vi "NF87XX.get start velocity.vi"(0 "i ref in":refnum<vi>, 2 "System":string="N/A", 5 "error in (no error)":errorcluster) -> (14 "i ref out":refnum<vi>, 16 "start velocity Mot 0 [Steps/s]":dbl, 17 "start velocity Mot 1 [Steps/s]":dbl, 18 "start velocity Mot 2 [Steps/s]":dbl, 19 "error out":errorcluster)   [LabVIEW 2014, in "NF87XX.lvlib"]
doc: "Gets the start velocity for all systems (drivers) and writes it to own attributes. Returns the start velocity of up to 3 motors in steps/s if \"System\" is found to be one of the driver names. Thereby 99999 indicates that an error occured or the value is not available.\n\nauthor: Stefan Götte\ndata: 09-JAN-2007\n\n\n\n\nLicense Agreement for this software:\n\nCopyright (C)\nGesellschaft für Schwerionenforschung, GSI\nPlanckstr. 1\n64291 Darmstadt\nGermany\n\nContact: D.Beck@gsi.de \n\nThis program is free software; you can redistribute it and/or modify it under the terms of the GNU General Public License as published by the Free Software Foundation; either version 2 of the license, or (at your option) any later version.\n\nThis program is distributed in the hope that it will be useful, but WITHOUT ANY WARRANTY; without even the implied warranty of MERCHANTABILITY or FITNESS FOR A PARTICULAR PURPOSE. See the GNU General License for more details (http://www.gnu.org).\n\nGesellschaft für Schwerionenforschung, GSI\nPlanckstr. 1, 64291 Darmstadt, Germany\nFor all questions and ideas contact: M.Richter@gsi.de, H.Brand@gsi.de or D.Beck@gsi.de.\nLast update: 17-JUN-2004"
uses:
  NF87XX.lvlib
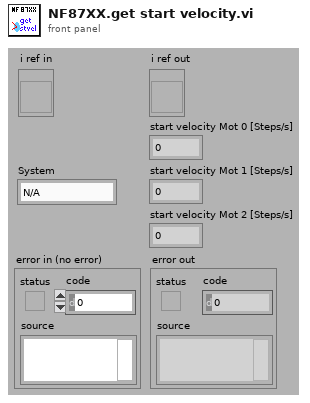
[diagram p1: front panel]
types:
  T1 = enum16{"User....", "DEF", "DIAG", "INI", "LOCK", "UNLOCK", "MAP", "SAV", "VER", "ACC", "CHL", "FOR", "GO", "HAL", "MOF", "MON", "MPV", "POS", "REL", "REV", "STA", "STO", "TYP", "VEL", "ABS", "SER", "NOS", "DRT", "FLI", "RLI", "FIN", "RIN", "AIN", "IN", "JOF", "JON", "OUT", "RES FINE", "RES COARSE", "02 (HEX)", "PWM", "CNT", "TMR", "HOSTNAME", "IPADDR", "IPMODE", "NETMASK", "GATEWAY", "DNSSRVR", "PASSWD", "ECHO", "MACADDR"}
  T2 = typedef "NF87XX.lvlib/NF87XX.driver Type.ctl" = enum16{"not defined", "3-ch open loop drv", "1-ch closed loop drv"}
  T3 = typedef "NF87XX.lvlib/NF87XX.i attribute.ctl" = cluster{"Con Settings":T4, "Drivers":T5[], "Status":cluster{"Service ID":i32, "Status":T7}, "Joystick available":bool, "VISA Resource":string}
  T4 = typedef "NewFocusPico - Driver np.lvlib/VISA & TCPIP Control.ctl" = cluster{"VISA or TCP/IP":bool, "Init Connection":bool, "Close Connection":bool, "Resource Name":refnum<visa-resource-name>, "hostname":string, "connection ID":refnum<k5>}
  T5 = typedef "NF87XX.lvlib/NF87XX.driver Settings.ctl" = cluster{"Name":string, "Driver Type":T2, "Pico Parameter type":T6, "Acceleration [Steps/s²]":cluster{"Motor 0":dbl, "Motor 1":dbl, "Motor 2":dbl}, "Start Velocity [Steps/s]":cluster{"Motor 0":dbl, "Motor 1":dbl, "Motor 2":dbl}, "Velocity [Steps/s]":cluster{"Motor 0":dbl, "Motor 1":dbl, "Motor 2":dbl}, "axis channel":i32, "Position":i32, "Position Service ID":i32}
  T6 = typedef "NewFocusPico - Driver np.lvlib/Pico Parameters.ctl" = cluster{"Pico Type":enum16{"Open-Loop Pico", "Close-Loop Pico", "Pico Ultra"}, "Acceleration (steps/sec^2)":string, "Velocity ( Hz)":string, "Driver":string, "Motor":string, "Channel":string, "Process Step":string}
  T7 = typedef "PH_StatusHandler.lvlib/PH_StatusHandler.Status.ctl" = i16
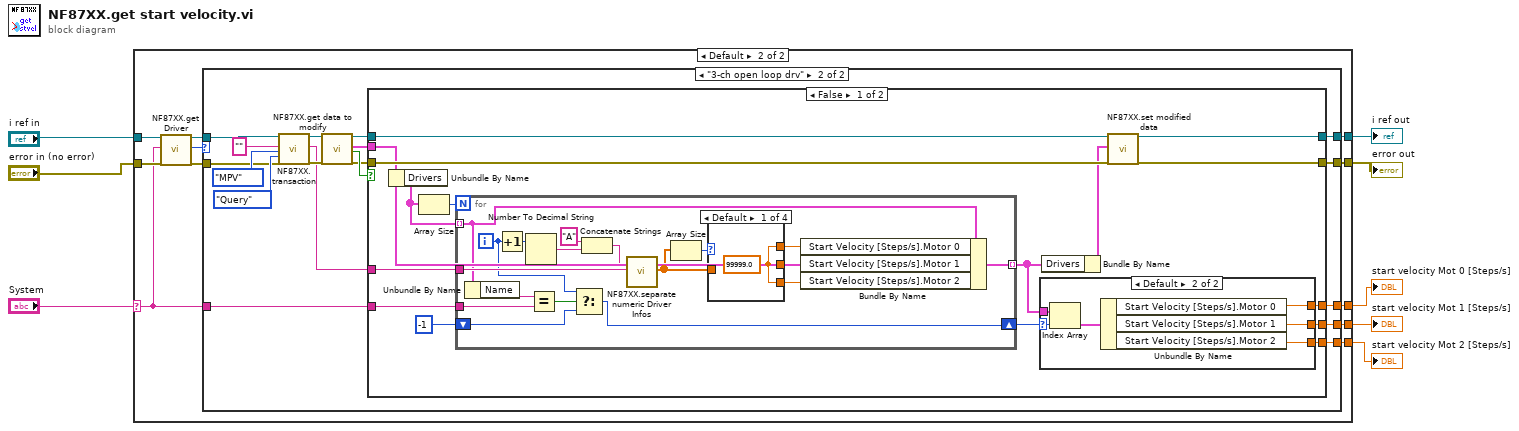
[diagram p0: block diagram]
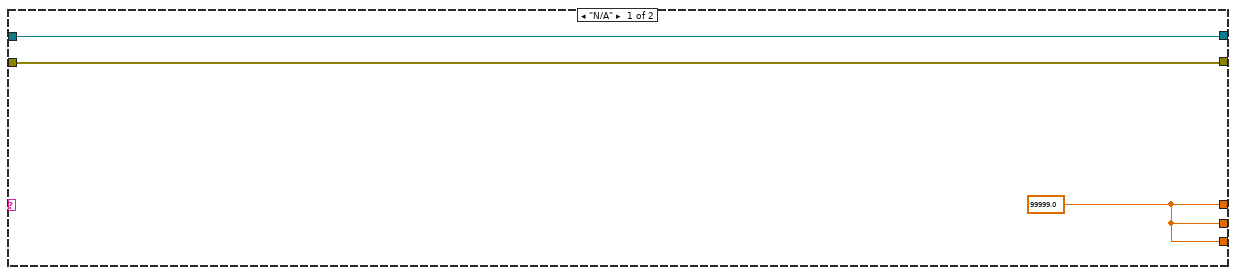
[diagram p2: hidden frame]
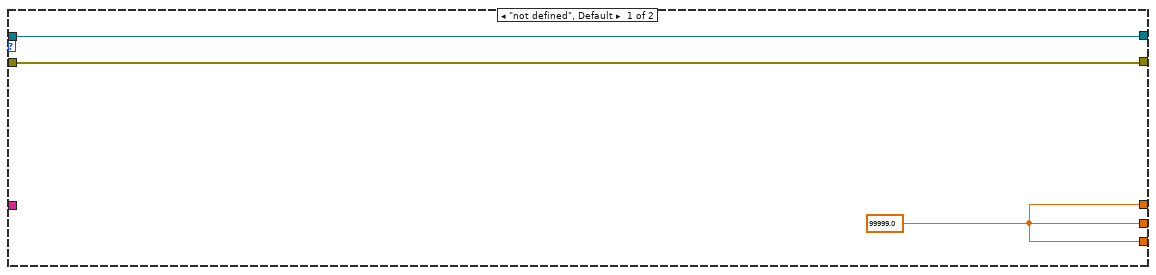
[diagram p3: hidden frame]
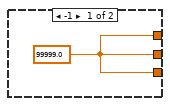
[diagram p4: hidden frame]
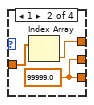
[diagram p5: hidden frame]
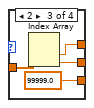
[diagram p6: hidden frame]
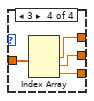
[diagram p7: hidden frame]
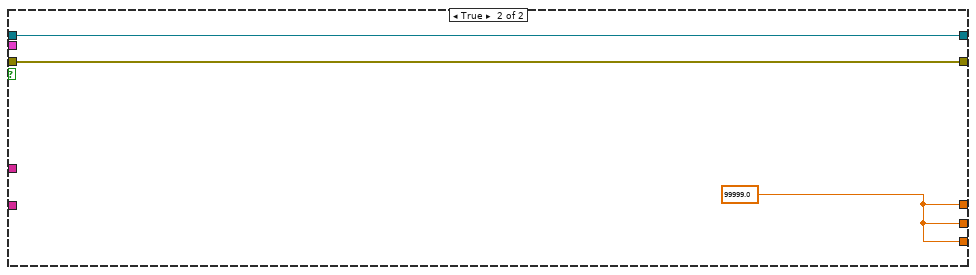
[diagram p8: hidden frame]
diagram:
  n1 = case shown="Default" "System" {
    selector: "System" -> [_ w13]
    tunnel: "error in (no error)" -> [w10 w15]
    tunnel: "i ref in" -> [w11 w17]
    tunnel: [w11 w22] -> w6
    tunnel: [w10 w21] -> w5
    tunnel: [w9 w20] -> w4
    tunnel: [w9 w19] -> w3
    tunnel: [w9 w18] -> w2
    frame "N/A" {
      w9 = 99999.0 ("Motor 0")
    }
    frame Default {
      n2 = call "NF87XX.get Driver.vi"("i ref in"=w17, "System"=w13, "error in (no error)"=w15) -> ("i ref out"=w16:refnum<vi>, "Driver Type"=w12:T2, "error out"=w14:errorcluster)  [unwired: 12 in, 2 out]
      n3 = case shown="\"3-ch open loop drv\"" w12 {
        tunnel: [w25 w33] -> w22
        tunnel: [w24 w32] -> w21
        tunnel: [w23 w31] -> w20
        tunnel: [w23 w30] -> w19
        tunnel: [w23 w29] -> w18
        tunnel: w16 -> [w25 w28]
        tunnel: w14 -> [w24 w27]
        tunnel: w13 -> [_ w26]
        frame "not defined", Default {
          w23 = 99999.0 ("Motor 0")
        }
        frame "3-ch open loop drv" {
          n4 = call "NF87XX.transaction.vi"("i ref in"=w28, "User Cmd/Numeric Argu"="", "MCL Cmd"=T1."MPV", "Query/Set"=enum16{"Query", "Set"}."Query", "error in (no error)"=w27) -> ("i ref out"=w35:refnum<vi>, "Read String"=w34:string, "error out"=w36:errorcluster)  [unwired: 12 in]
          n5 = call "NF87XX.get data to modify.vi"("i ref in"=w35, "error in (no error)"=w36) -> ("i ref out"=w39:refnum<vi>, "i attribute"=w38:T3, "timed out"=w40:bool, "error out"=w37:errorcluster)  [unwired: 14 in]
          n6 = case shown="False" w40 {
            tunnel: w39 -> [w59 w99]
            tunnel: w38 -> [w53 _]
            tunnel: [w56 w99] -> w33
            tunnel: w37 -> [w58 w98]
            tunnel: [w57 w98] -> w32
            tunnel: w34 -> [w55 _]
            tunnel: w26 -> [w50 _]
            tunnel: [w47 w97] -> w31
            tunnel: [w46 w97] -> w30
            tunnel: [w45 w97] -> w29
            frame False {
              n7 = Unbundle By Name(w53) -> ("Drivers"=w49:T5[])
              n8 = Array Size(array=w49) -> (size(s)=w54:i32)
              n9 = for {
                N: w54 -> [_]
                tunnel: w55 -> [w84]
                tunnel: w49 -> [w68] mode=indexing
                tunnel: [w67] -> w51 mode=indexing
                tunnel: w50 -> [w75]
                shift-right: [w76] -> w44
                shift-left: -1 -> [w72]
                i -> [w73]
                n10 = Unbundle By Name(w68) -> ("Name"=w74:string)
                n11 = Increment(x=w73) -> (x+1=w83:i32)
                n12 = Number To Decimal String(number=w83) -> (decimal integer string=w81:string)  [unwired: 1 in]
                n13 = Equal?(x=w74, y=w75) -> (x = y?=w77:bool)
                n14 = Select(t=w73, s=w77, f=w72) -> (s? t:f=w76:i32)
                n15 = Concatenate Strings("A" ("string"), w81) -> (w80:string)
                n16 = call "NF87XX.separate numeric Driver Infos.vi"("Driver"=w80, "Read String"=w84) -> ("Result"=w78:dbl[])  [unwired: 17 in]
                n17 = Array Size(array=w78) -> (size(s)=w79:i32)
                n18 = case shown="Default" w79 {
                  tunnel: w78 -> [_ w88 w92 w96]
                  tunnel: [w85 w87 w91 w95] -> w71
                  tunnel: [w85 w86 w90 w94] -> w70
                  tunnel: [w85 w86 99999.0 w93] -> w69
                  frame Default {
                    w85 = 99999.0
                  }
                  frame 1 {
                    w86 = 99999.0
                    n19 = Index Array(array=w88) -> (element=w87:dbl)  [unwired: 1 in]
                  }
                  frame 2 {
                    n20 = Index Array(array=w92) -> (element #1=w91:dbl, element #2=w90:dbl)  [unwired: 2 in]
                  }
                  frame 3 {
                    n21 = Index Array(array=w96) -> (element #1=w95:dbl, element #2=w94:dbl, element #3=w93:dbl)  [unwired: 3 in]
                  }
                }
                n22 = Bundle By Name(cluster=w68, "Start Velocity [Steps/s].Motor 0"=w71, "Start Velocity [Steps/s].Motor 1"=w70, "Start Velocity [Steps/s].Motor 2"=w69) -> (w67:T5)
              }
              n23 = case shown="Default" w44 {
                selector: w44 -> [_ w61]
                tunnel: w51 -> [_ w66]
                tunnel: [w60 w64] -> w47
                tunnel: [w60 w63] -> w46
                tunnel: [w60 w62] -> w45
                frame -1 {
                  w60 = 99999.0 ("Motor 1")
                }
                frame Default {
                  n24 = Index Array(array=w66, index=w61) -> (element=w65:T5)
                  n25 = Unbundle By Name(w65) -> ("Start Velocity [Steps/s].Motor 0"=w64:dbl, "Start Velocity [Steps/s].Motor 1"=w63:dbl, "Start Velocity [Steps/s].Motor 2"=w62:dbl)
                }
              }
              n26 = Bundle By Name(cluster=w53, "Drivers"=w51) -> (w52:T3)
              n27 = call "NF87XX.set modified data.vi"("i ref in"=w59, "i attribute"=w52, "error in (no error)"=w58) -> ("i ref out"=w56:refnum<vi>, "error out"=w57:errorcluster)  [unwired: 15 in]
            }
            frame True {
              w97 = 99999.0 ("Motor 0")
            }
          }
        }
      }
    }
  }
  "error out" <- w5
  "i ref out" <- w6
  "start velocity Mot 0 [Steps/s]" <- w4
  "start velocity Mot 1 [Steps/s]" <- w3
  "start velocity Mot 2 [Steps/s]" <- w2
